vi "Car Wash.vi"() -> ()   [LabVIEW 2023]
uses:
  Controls/Car Wash Indicators.ctl
  Controls/Wash Options.ctl
  Controls/Queued_Data.ctl
  Controls/State.ctl
  Controls/System_Data.ctl
  Controls/User_Event.ctl
  Controls/Producer_Cluster.ctl
  199d70cd-2b2d-4eda-8243-a0dbe1aab652.vi
panel:
  out "error out":errorcluster
  in  "error in":errorcluster
  in  "Start":bool
  out "Elapsed Time":dbl format="%0.2f"
  in  "stop":bool
  out "Wash Entry":bool
  in  "Wash Options":T1
  in  "Car Position Slider":u8(slide) max=3 scale=0.0..4.0
  out "Car Wash Indicators":T2
  # "Car Wash Display"
  # "Entry Console"
  # "Car Position Simulation"
  # "Pre-Soak\nH-P Wash\nL-P Wax\nSpot Free Rinse"
  # "Underbody Wash\nBug Remover"
  # "Tire Shine\nAir Dry"
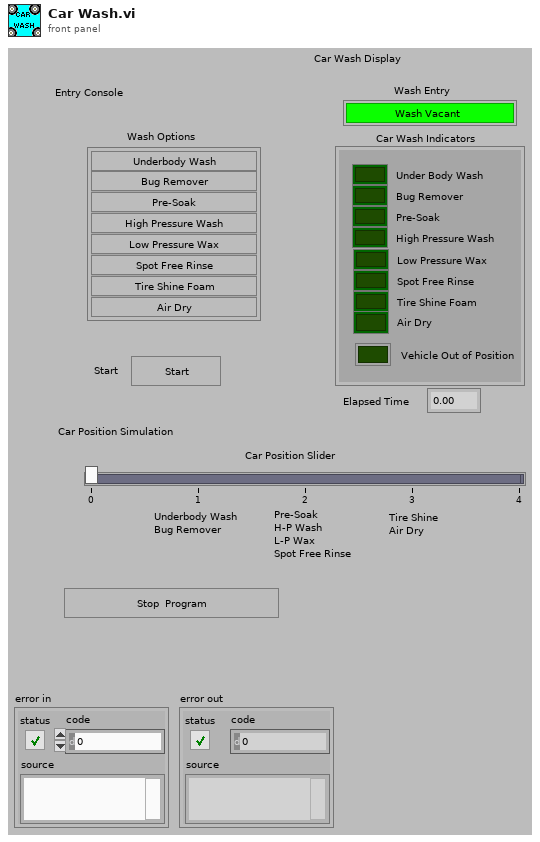
[diagram p1: front panel]
types:
  T1 = typedef "Wash Options.ctl" = cluster{"Underbody Wash":bool, "Bug Remover":bool, "Pre-Soak":bool, "High Pressure Wash":bool, "Low Pressure Wax":bool, "Spot Free Rinse":bool, "Tire Shine Foam":bool, "Air Dry":bool}
  T2 = typedef "Car Wash Indicators.ctl" = cluster{"Under Body Wash":bool, "Bug Remover":bool, "Pre-Soak":bool, "High Pressure Wash":bool, "Low Pressure Wax":bool, "Spot Free Rinse":bool, "Tire Shine Foam":bool, "Air Dry":bool, "Vehicle Out of Position":bool}
  T3 = typedef "Producer_Cluster.ctl" = cluster{"Step Time":dbl, "Reset":bool, "Pause":bool, "Elapsed Time":dbl}
  T4 = typedef "State.ctl" = enum16{"Initialize", "Wait for Something", "Step Completed", "Save Wash Options", "Start Process", "Car Position", "Order Steps to follow", "Underbody Wash", "Bug Remover", "Pre-Soak", "High Pressure Wash", "Low Pressure Wax", "Spot Free Rinse", "Tire Shine Foam", "Air Dry", "Vehicle out of position", "Exit", "Process Complete", "Stop Application"}
  T5 = typedef "User_Event.ctl" = cluster{"Step Time":dbl, "Timeout":i32, "Pause":bool}
  T6 = enum8{"Enabled", "Disabled", "Disabled and Grayed Out"}
  T7 = typedef "System_Data.ctl" = cluster{"Start button":bool, "Wash Options":T1, "Enabled Steps Index":i32[], "Enabled Steps ":T4[], "Index Current Step":i32, "Car Position":u8, "Step Time":dbl[], "Timeout":i32, "Timer started":bool, "Paused":bool}
  T8 = typedef "Queued_Data.ctl" = cluster{"State":T4, "Data":variant}
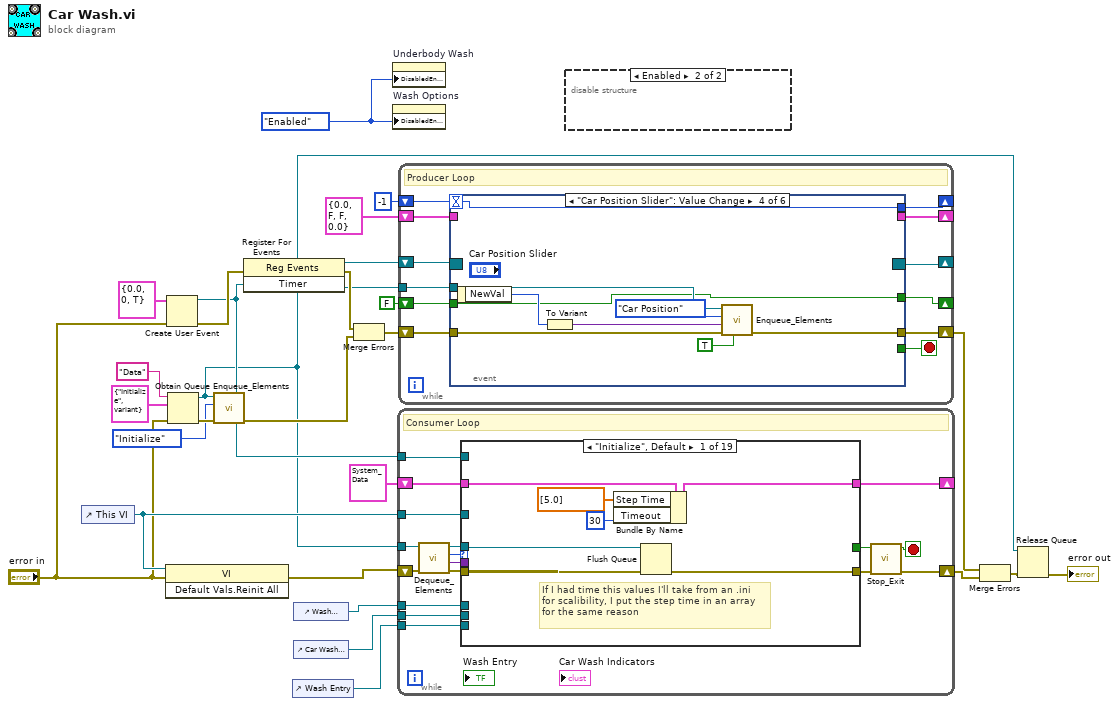
[diagram p0: block diagram]
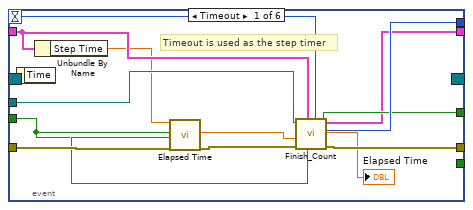
[diagram p2: hidden frame]
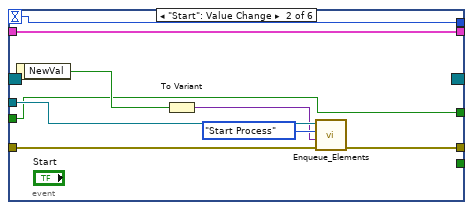
[diagram p3: hidden frame]
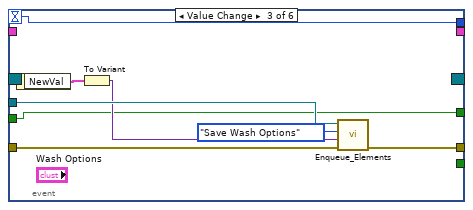
[diagram p4: hidden frame]
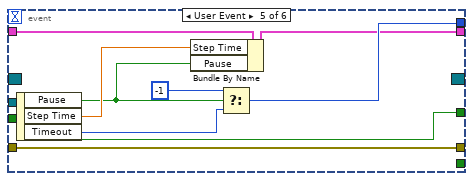
[diagram p5: hidden frame]
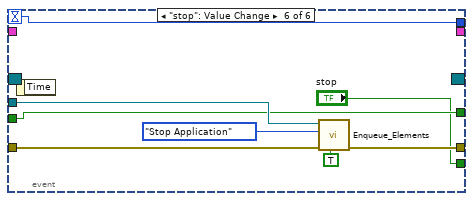
[diagram p6: hidden frame]
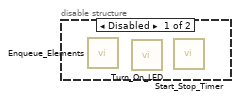
[diagram p7: hidden frame]
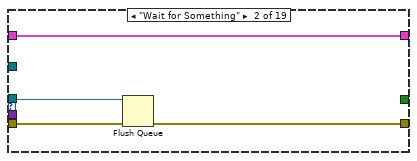
[diagram p8: hidden frame]
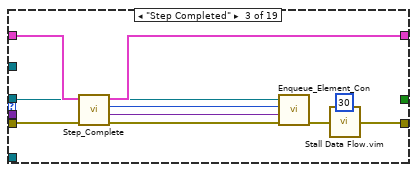
[diagram p9: hidden frame]
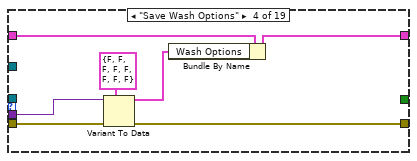
[diagram p10: hidden frame]
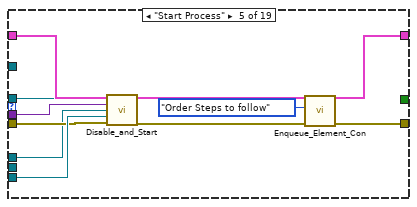
[diagram p11: hidden frame]
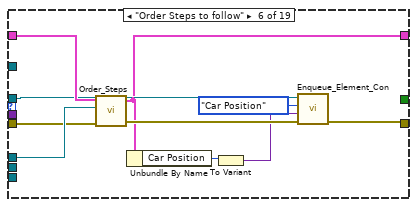
[diagram p12: hidden frame]
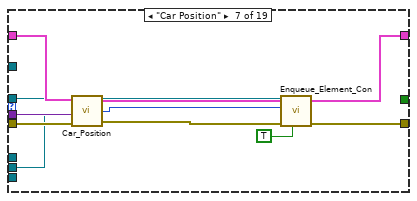
[diagram p13: hidden frame]
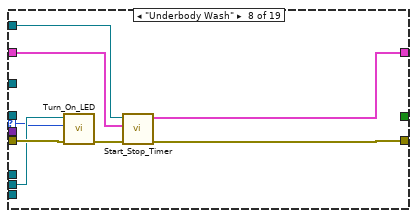
[diagram p14: hidden frame]
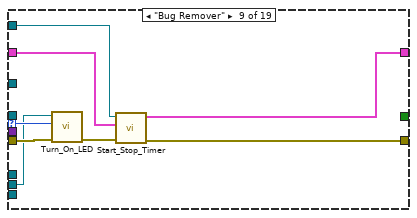
[diagram p15: hidden frame]
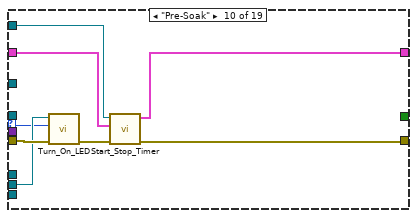
[diagram p16: hidden frame]
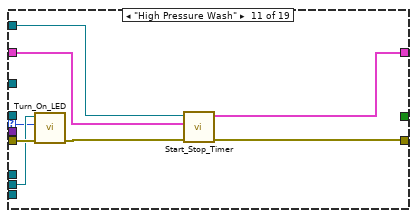
[diagram p17: hidden frame]
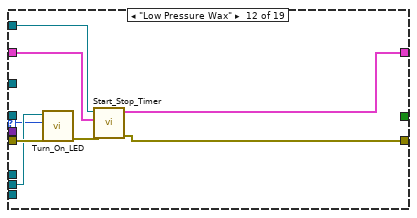
[diagram p18: hidden frame]
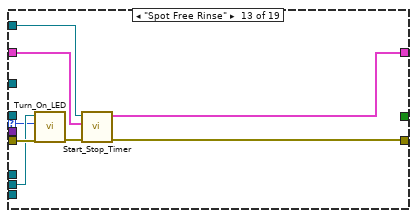
[diagram p19: hidden frame]
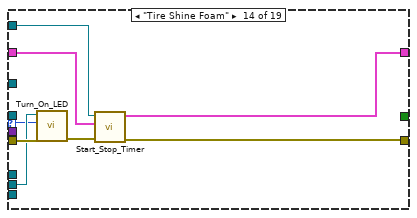
[diagram p20: hidden frame]
diagram:
  w19 = T6."Enabled" ("Disabled")
  n1 = control-ref of="This VI"() -> (w18:refnum<vi>)
  n2 = invoke class="VI" method="Default Vals.Reinit All"(reference=w18, error in="error in") -> (error out=w17:errorcluster)  [unwired: 1 in, 2 out]
  n3 = Create User Event(user event datatype=T5 {"Step Time"=0.0, "Timeout"=0, "Pause"=TRUE} ("Timer"), error in="error in") -> (user event=w10:refnum<user-event>, error out=w12:errorcluster)
  n4 = Obtain Queue(name (unnamed)="Data", element data type=T8 {"State"=enum."Initialize", "Data"=variant}, error in (no error)="error in") -> (queue out=w3:refnum<queue>, error out=w6:errorcluster)  [unwired: 2 in, 1 out]
  n5 = call "Enqueue_Elements.vi"("error in (no error)"=w6, "State"=State."Initialize", "Queue in"=w3) -> ("error out"=w5:errorcluster)  [unwired: 8 in]
  n6 = register-events(error in=w12, w10) -> (reference out=w11:refnum<event-registration>, error out=w13:errorcluster)  [unwired: 1 in]
  n7 = control-ref of="Wash Entry"() -> (w21:refnum<vi>)
  n8 = control-ref of="Wash Options"() -> (w20:refnum<vi>)
  n9 = control-ref of="Car Wash Indicators"() -> (w22:refnum<vi>)
  n10 = Merge Errors(w13, w5) -> (w15:errorcluster)
  n11 = property on="Underbody Wash" class="Bool (strict)"("DisabledEnum"=w19) -> ()  [unwired: 2 in, 2 out]
  n12 = property on="Wash Options" class="Clust (strict)"("DisabledEnum"=w19) -> ()  [unwired: 2 in, 2 out]
  n13 = while {
    shift-right: [w42] -> w26
    shift-left: w17 -> [w28]
    tunnel: w3 -> [w40]
    shift-right: [w37] -> _
    shift-left: T7 {"Start button"=FALSE, "Wash Options"={"Underbody Wash"=FALSE, "Bug Remover"=FALSE, "Pre-Soak"=FALSE, "High Pressure Wash"=FALSE, "Low Pressure Wax"=FALSE, "Spot Free Rinse"=FALSE, "Tire Shine Foam"=FALSE, "Air Dry"=FALSE}, "Enabled Steps Index"=[], "Enabled Steps "=[], "Index Current Step"=0, "Car Position"=0, "Step Time"=[], "Timeout"=0, "Timer started"=FALSE, "Paused"=FALSE} -> [w38]
    tunnel: w20 -> [w35]
    tunnel: w22 -> [w31]
    tunnel: w21 -> [w34]
    tunnel: w18 -> [w33]
    tunnel: w10 -> [w29]
    stop <- w44 stop-if-true
    # "Consumer Loop"
    n14 = call "Dequeue_Elements.vi"("error in (no error)"=w28, "Queue in"=w40) -> ("error out"=w41:errorcluster, "Data"=w39:variant, "State"=w30:T4, "queue out"=w36:refnum<queue>)  [unwired: 2 in]
    n15 = case shown="\"Initialize\", Default" w30 {
      selector: w30 -> [_ _ _ _ _ _ _ w108 w118 w124 w132 w140 w148 w156 w164 _ _ _ _]
      tunnel: w41 -> [w51 w55 w57 w72 w75 w90 w102 w110 w117 w126 w134 w142 w150 w158 w166 w175 w183 w186 w192]
      tunnel: [w46 w53 w59 w70 w73 w88 w98 w106 w114 w122 w130 w138 w146 w154 w162 w177 w182 w185 w194] -> w43
      tunnel: w39 -> [_ _ _ w69 w81 _ w100 _ _ _ _ _ _ _ _ _ _ _ _]
      tunnel: w38 -> [w50 w54 w65 w71 w82 w92 w101 w105 w113 w121 w129 w137 w145 w153 w161 w171 w180 w187 w195]
      tunnel: [w49 w54 w64 w67 w80 w85 w99 w103 w111 w119 w127 w135 w143 w151 w159 w170 w178 w187 w195] -> w37
      tunnel: w36 -> [w45 w52 w62 _ w78 w87 w96 _ _ _ _ _ _ _ _ w168 _ w184 _]
      tunnel: w35 -> [_ _ _ _ w74 w91 _ _ _ _ _ _ _ _ _ w172 _ _ w191]
      tunnel: w31 -> [_ _ _ _ _ _ w93 w109 w116 w125 w133 w141 w149 w157 w165 _ w179 _ _]
      tunnel: w34 -> [_ _ _ _ w76 _ _ _ _ _ _ _ _ _ _ _ _ _ w189]
      tunnel: w33 -> [_ _ _ _ _ _ _ _ _ _ _ _ _ _ _ w173 _ _ w193]
      tunnel: [_ _ _ _ _ _ _ _ _ _ _ _ _ _ _ _ _ _ TRUE] -> w32
      tunnel: w29 -> [_ _ _ _ _ _ _ w104 w112 w120 w128 w136 w144 w152 w160 _ w181 _ _]
      frame "Initialize", Default {
        # "If I had time this values I'll take from an .ini\nfor scalibility, I put the step time in an array\nfor the same reason"
        n16 = Bundle By Name(cluster=w50, "Step Time"=dbl[] [5.0], "Timeout"=30) -> (w49:T7)
        n17 = Flush Queue(queue=w45, error in (no error)=w51) -> (error out=w46:errorcluster)  [unwired: 2 out]
      }
      frame "Wait for Something" {
        n18 = Flush Queue(queue=w52, error in (no error)=w55) -> (error out=w53:errorcluster)  [unwired: 2 out]
      }
      frame "Step Completed" {
        n19 = call "Step_Complete.vi"("error in"=w57, "System data in"=w65) -> ("error out"=w56:errorcluster, "Car Position"=w61:variant, "State"=w60:T4, "System data out"=w64:T7)  [unwired: 6 in]
        n20 = call "Enqueue_Element_Con.vi"("error in (no error)"=w56, "Data"=w61, "State"=w60, "Queue in"=w62) -> ("error out"=w63:errorcluster)  [unwired: 7 in]
        n21 = call "Stall Data Flow.vim"("value in"=w63, "milliseconds to wait"=u32 30) -> ("value out"=w59:errorcluster)  [unwired: 1 out]
      }
      frame "Save Wash Options" {
        n22 = Variant To Data(error in=w72, type=T1 {"Underbody Wash"=FALSE, "Bug Remover"=FALSE, "Pre-Soak"=FALSE, "High Pressure Wash"=FALSE, "Low Pressure Wax"=FALSE, "Spot Free Rinse"=FALSE, "Tire Shine Foam"=FALSE, "Air Dry"=FALSE} ("Wash Options"), Variant=w69) -> (data=w66:T1, error out=w70:errorcluster)
        n23 = Bundle By Name(cluster=w71, "Wash Options"=w66) -> (w67:T7)
      }
      frame "Start Process" {
        n24 = call "Disable_and_Start.vi"("System data in"=w82, "Data"=w81, "Wash Options In"=w74, "Wash Entry"=w76, "error in (no error)"=w75) -> ("System data out"=w80:T7, "error out"=w79:errorcluster)  [unwired: 9 in]
        n25 = call "Enqueue_Element_Con.vi"("error in (no error)"=w79, "State"=State."Order Steps to follow", "Queue in"=w78) -> ("error out"=w73:errorcluster)  [unwired: 8 in]
      }
      frame "Order Steps to follow" {
        n26 = call "Order_Steps.vi"("System data"=w92, "Wash Options"=w91, "error in (no error)"=w90) -> ("System data out"=w85:T7, "error out"=w89:errorcluster)  [unwired: 3 in]
        n27 = Unbundle By Name(w85) -> ("Car Position"=w84:u8)
        n28 = To Variant(anything=w84) -> (Variant=w83:variant)
        n29 = call "Enqueue_Element_Con.vi"("error in (no error)"=w89, "Data"=w83, "State"=State."Car Position", "Queue in"=w87) -> ("error out"=w88:errorcluster)  [unwired: 7 in]
      }
      frame "Car Position" {
        n30 = call "Car_Position.vi"("error in (no error)"=w102, "Car Wash Indicators"=w93, "Data"=w100, "System data in"=w101) -> ("error out"=w97:errorcluster, "State"=w95:T4, "System data out"=w99:T7)
        n31 = call "Enqueue_Element_Con.vi"("Prioritize?"=TRUE, "error in (no error)"=w97, "State"=w95, "Queue in"=w96) -> ("error out"=w98:errorcluster)  [unwired: 7 in]
      }
      frame "Underbody Wash" {
        n32 = call "Turn_On_LED.vi"("error in (no error)"=w110, "State"=w108, "Car Wash Indicators"=w109) -> ("error out"=w107:errorcluster)  [unwired: 8 in]
        n33 = call "Start_Stop_Timer.vi"("error in (no error)"=w107, "System data"=w105, "user event in"=w104) -> ("error out"=w106:errorcluster, "System data out"=w103:T7)  [unwired: 7 in]
      }
      frame "Bug Remover" {
        n34 = call "Turn_On_LED.vi"("error in (no error)"=w117, "State"=w118, "Car Wash Indicators"=w116) -> ("error out"=w115:errorcluster)  [unwired: 8 in]
        n35 = call "Start_Stop_Timer.vi"("error in (no error)"=w115, "System data"=w113, "user event in"=w112) -> ("error out"=w114:errorcluster, "System data out"=w111:T7)  [unwired: 7 in]
      }
      frame "Pre-Soak" {
        n36 = call "Turn_On_LED.vi"("error in (no error)"=w126, "State"=w124, "Car Wash Indicators"=w125) -> ("error out"=w123:errorcluster)  [unwired: 8 in]
        n37 = call "Start_Stop_Timer.vi"("error in (no error)"=w123, "System data"=w121, "user event in"=w120) -> ("error out"=w122:errorcluster, "System data out"=w119:T7)  [unwired: 7 in]
      }
      frame "High Pressure Wash" {
        n38 = call "Turn_On_LED.vi"("error in (no error)"=w134, "State"=w132, "Car Wash Indicators"=w133) -> ("error out"=w131:errorcluster)  [unwired: 8 in]
        n39 = call "Start_Stop_Timer.vi"("error in (no error)"=w131, "System data"=w129, "user event in"=w128) -> ("error out"=w130:errorcluster, "System data out"=w127:T7)  [unwired: 7 in]
      }
      frame "Low Pressure Wax" {
        n40 = call "Turn_On_LED.vi"("error in (no error)"=w142, "State"=w140, "Car Wash Indicators"=w141) -> ("error out"=w139:errorcluster)  [unwired: 8 in]
        n41 = call "Start_Stop_Timer.vi"("error in (no error)"=w139, "System data"=w137, "user event in"=w136) -> ("error out"=w138:errorcluster, "System data out"=w135:T7)  [unwired: 7 in]
      }
      frame "Spot Free Rinse" {
        n42 = call "Turn_On_LED.vi"("error in (no error)"=w150, "State"=w148, "Car Wash Indicators"=w149) -> ("error out"=w147:errorcluster)  [unwired: 8 in]
        n43 = call "Start_Stop_Timer.vi"("error in (no error)"=w147, "System data"=w145, "user event in"=w144) -> ("error out"=w146:errorcluster, "System data out"=w143:T7)  [unwired: 7 in]
      }
      frame "Tire Shine Foam" {
        n44 = call "Turn_On_LED.vi"("error in (no error)"=w158, "State"=w156, "Car Wash Indicators"=w157) -> ("error out"=w155:errorcluster)  [unwired: 8 in]
        n45 = call "Start_Stop_Timer.vi"("error in (no error)"=w155, "System data"=w153, "user event in"=w152) -> ("error out"=w154:errorcluster, "System data out"=w151:T7)  [unwired: 7 in]
      }
      frame "Air Dry" {
        n46 = call "Turn_On_LED.vi"("error in (no error)"=w166, "State"=w164, "Car Wash Indicators"=w165) -> ("error out"=w163:errorcluster)  [unwired: 8 in]
        n47 = call "Start_Stop_Timer.vi"("error in (no error)"=w163, "System data"=w161, "user event in"=w160) -> ("error out"=w162:errorcluster, "System data out"=w159:T7)  [unwired: 7 in]
      }
      frame "Exit" {
        n48 = Flush Queue(queue=w168) -> (queue out=w167:refnum<queue>)  [unwired: 1 in, 2 out]
        n49 = call "Reinit_Default.vi"("error in (no error)"=w175, "System data in"=w171, "Wash Options"=w172, "VI in"=w173) -> ("error out"=w174:errorcluster, "System data out"=w170:T7)  [unwired: 6 in]
        n50 = call "Enqueue_Element_Con.vi"("Prioritize?"=TRUE, "error in (no error)"=w174, "State"=State."Process Complete", "Queue in"=w167) -> ("error out"=w177:errorcluster)  [unwired: 7 in]
      }
      frame "Vehicle out of position" {
        n51 = call "Out_of_Position.vi"("error in (no error)"=w183, "Car Wash Indicators"=w179, "System data"=w180, "Timer"=w181) -> ("error out"=w182:errorcluster, "System data out"=w178:T7)  [unwired: 6 in]
      }
      frame "Process Complete" {
        n52 = Flush Queue(queue=w184, error in (no error)=w186) -> (error out=w185:errorcluster)  [unwired: 2 out]
      }
      frame "Stop Application" {
        n53 = control-ref of="Car Position"() -> (w190:refnum<vi>)
        n54 = call "Stop_App.vi"("Wash Entry"=w189, "error in (no error)"=w192, "Wash Options"=w191, "This VI"=w193, "Car Position"=w190) -> ("error out"=w194:errorcluster)  [unwired: 6 in]
      }
    }
    n55 = call "Stop_Exit.vi"("error in (no error)"=w43, "STOP button"=w32) -> ("error out"=w42:errorcluster, "Exit While"=w44:bool)  [unwired: 8 in]
  }
  n56 = while {
    tunnel: w3 -> [w207]
    shift-right: [w205] -> w14
    shift-left: w15 -> [w206]
    shift-right: [w203] -> _
    shift-left: w11 -> [w204]
    shift-right: [w201] -> _
    shift-left: -1 -> [w202]
    shift-right: [w199] -> _
    shift-left: FALSE -> [w200]
    shift-right: [w197] -> _
    shift-left: T3 {"Step Time"=0.0, "Reset"=FALSE, "Pause"=FALSE, "Elapsed Time"=0.0} -> [w198]
    stop <- w196 stop-if-true
    # "Producer Loop"
    n57 = event shown="[3] \"Car Position Slider\": Value Change" {
      selector: w204 -> [_ _ _ _ _ _]
      dyn-events: [_ _ _ _ _ _] -> w203
      timeout: w202 -> [w218 w224 w232 w240 _ w259]
      tunnel: w207 -> [w214 w230 w236 w247 _ w263]
      tunnel: w206 -> [w221 w229 w237 w243 w256 w261]
      tunnel: [w216 w228 w238 w245 w256 w264] -> w205
      tunnel: [w219 w224 w232 w240 w253 w259] -> w201
      tunnel: w200 -> [w213 w223 w231 w239 w255 w258]
      tunnel: [w212 w223 w231 w239 w255 w258] -> w199
      tunnel: w198 -> [w211 w222 _ _ w251 _]
      tunnel: [w209 w222 _ _ w250 _] -> w197
      tunnel: [_ _ _ _ _ "stop"] -> w196
      event Timeout {
        # "Timeout is used as the step timer"
        n58 = event-data() -> ()  [unwired: 1 in, 1 out]
        n59 = Unbundle By Name(w211) -> ("Step Time"=w210:dbl)
        n60 = call "Elapsed Time"("Time Target (s)"=w210, "Reset"=w213, "Auto Reset"=w213, "error in (no error)"=w221) -> ("Elapsed Time (s)"=w215:dbl, "Time has Elapsed"=w220:bool, "error out"=w217:errorcluster)  [unwired: 8 in, 5 out]
        n61 = call "Finish_Count"("Timeout"=w218, "Time has Elapsed"=w220, "Producer Cluster in"=w211, "error in (no error)"=w217, "Elapsed Time (s) in"=w215, "Queue in"=w214) -> ("error out"=w216:errorcluster, "Time Elapsed"=w212:bool, "Timeout"=w219:i32, "Producer Cluster out"=w209:T3, "Elapsed Time (s) out"=→"Elapsed Time":dbl)  [unwired: 1 in]
      }
      event "Start": Value Change {
        n62 = event-data() -> ("NewVal"=w226:bool)  [unwired: 1 in]
        n63 = To Variant(anything=w226) -> (Variant=w225:variant)
        n64 = call "Enqueue_Elements.vi"("error in (no error)"=w229, "Data"=w225, "State"=State."Start Process", "Queue in"=w230) -> ("error out"=w228:errorcluster)  [unwired: 7 in]
      }
      event Value Change {
        n65 = event-data() -> ("NewVal"=w235:T1)  [unwired: 1 in]
        n66 = To Variant(anything=w235) -> (Variant=w233:variant)
        n67 = call "Enqueue_Elements.vi"("error in (no error)"=w237, "Data"=w233, "State"=State."Save Wash Options", "Queue in"=w236) -> ("error out"=w238:errorcluster)  [unwired: 7 in]
      }
      event "Car Position Slider": Value Change {
        n68 = event-data() -> ("NewVal"=w246:u8)  [unwired: 1 in]
        n69 = To Variant(anything=w246) -> (Variant=w242:variant)
        n70 = call "Enqueue_Elements.vi"("Prioritize?"=TRUE, "error in (no error)"=w243, "Data"=w242, "State"=State."Car Position", "Queue in"=w247) -> ("error out"=w245:errorcluster)  [unwired: 6 in]
      }
      event User Event {
        n71 = event-data() -> ("Pause"=w248:bool, "Step Time"=w249:dbl, "Timeout"=w254:i32)  [unwired: 1 in]
        n72 = Bundle By Name(cluster=w251, "Step Time"=w249, "Pause"=w248) -> (w250:T3)
        n73 = Select(t=-1, s=w248, f=w254) -> (s? t:f=w253:i32)
      }
      event "stop": Value Change {
        n74 = event-data() -> ()  [unwired: 1 in, 1 out]
        n75 = call "Enqueue_Elements.vi"("Prioritize?"=TRUE, "error in (no error)"=w261, "State"=State."Stop Application", "Queue in"=w263) -> ("error out"=w264:errorcluster)  [unwired: 7 in]
      }
    }
  }
  n76 = disable-structure shown="Enabled" {
    frame Disabled {
      n77 = call "Enqueue_Elements.vi"() -> ()  [unwired: 11 in, 1 out]
      n78 = call "Turn_On_LED.vi"() -> ()  [unwired: 11 in, 1 out]
      n79 = call "Start_Stop_Timer.vi"() -> ()  [unwired: 10 in, 2 out]
    }
    frame Enabled {
    }
  }
  n80 = Merge Errors(w14, w26) -> (w16:errorcluster)
  n81 = Release Queue(queue=w3, error in (no error)=w16) -> (error out=→"error out":errorcluster)  [unwired: 1 in, 2 out]
